vi "Get Error (Scope).vi"(8 "error in (no error)":errorcluster, 10 "scope":T1, 11 "error list <top>":variant) -> (0 "error out":errorcluster, 1 "found?":bool, 2 "error list <scope>":variant, 3 "error list <top> dup":variant)   [LabVIEW 2017]
uses:
  Scope.ctl
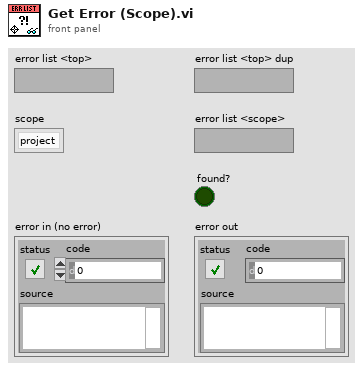
[diagram p1: front panel]
types:
  T1 = typedef "Scope.ctl" = enum16{"project", "global"}
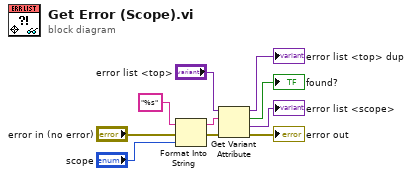
[diagram p0: block diagram]
diagram:
  n1 = Format Into String(format string="%s", error in="error in (no error)", "scope") -> (resulting string=w8:string, error out=w9:errorcluster)  [unwired: 1 in]
  n2 = Get Variant Attribute(Variant="error list <top>", name=w8, error in=w9) -> (duplicate Variant=→"error list <top> dup":variant, found=→"found?":bool, value=→"error list <scope>":variant, error out=→"error out":errorcluster)  [unwired: 1 in]
